vi "init.vi"(0 "Camera in":refnum<class "Camera.lvclass">, 1 "interface":u8(ring)=255 items=["FireWire"=1, "GenICam"=3, "GigE"=5, "USB"=6, "CameraLinkME4"=7, "USB3"=8, "CLHS"=11, "All"=255], 3 "error in (no error)":errorcluster) -> (7 "Camera out":refnum<class "Camera.lvclass">, 10 "error out":errorcluster)   [LabVIEW 2020, in "Camera.lvclass"]
doc: "This function is similar to init.vi but with the additional option to select the interface where\ncameras should be searched for. The default is All Interfaces. In contrast to init.vi, this function\nuses the pco.sdk function PCO_OpenCameraEx.vi to search the interfaces individually.\n\nYou should use this function instead of init.vi when:\n - You want to search for cameras at a specific interface.\n - You want to create multiple Camera objects in an application where the cameras are partially connected during operation."
uses:
  Camera.lvclass
  Camera.lvclass/Camera.ctl
  Structures.lvlib
  CameraAccess.lvlib
  CameraDescription.lvlib
  GeneralCameraStatus.lvlib
  Convert.lvlib
panel:
  out "error out 2":errorcluster {"code" format="%x"}
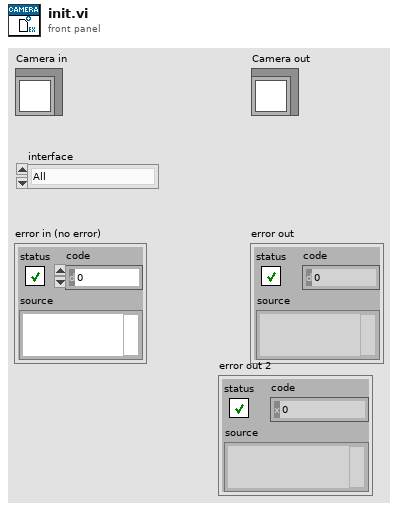
[diagram p1: front panel]
types:
  T1 = cluster{"wCamType":u16, "wCamSubType":u16, "dwSerialNumber":u32, "dwHWVersion":u32, "dwFWVersion":u32, "InterfaceType":u16, "PCO_FW_Vers":cluster{"wDeviceNum":u16, "PCO_SC2_Firmware_DESC":cluster{"szName":string, "bMinorRev":u8, "bMajorRev":u8, "wVariant":u16}[]}, "PCO_HW_Vers":cluster{"wBoardNum":u16, "PCO_SC2_Hardware_DESC":cluster{"szName":string, "wBatchNo":u16, "wRevision":u16, "wVariant":u16}[]}}
  T2 = cluster{"wSensorTypeDESC":u16, "wSensorSubTypeDESC":u16, "wMaxHorzResStdDESC":u16, "wMaxVertResStdDESC":u16, "wMaxHorzResExtDESC":u16, "wMaxVertResExtDESC":u16, "wDynResDESC":u16, "wMaxBinHorzDESC":u16, "wBinHorzSteppingDESC":u16, "wMaxBinVertDESC":u16, "wBinVertSteppingDESC":u16, "wRoiHorStepsDESC":u16, "wRoiVertStepsDESC":u16, "wNumADCsDESC":u16, "wMinSizeHorzDESC":u16, "dwPixelRateDESC":u32[], "wConvFactDESC":u16[], "sCoolingSetpoints":i16[], "wSoftRoiHorStepsDESC":u16, "wSoftRoiVertStepsDESC":u16, "wIRDESC":u16, "wMinSizeVertDESC":u16, "dwMinDelayDESC":u32, "dwMaxDelayDESC":u32, "dwMinDelayStepDESC":u32, "dwMinExposureDESC":u32, "dwMaxExposureDESC":u32, "dwMinExposureStepDESC":u32, "dwMinDelayIRDESC":u32, "dwMaxDelayIRDESC":u32, "dwMinExposureIRDESC":u32, "dwMaxExposureIRDESC":u32, "wTimeTableDESC":u16, "wDoubleImageDESC":u16, "sMinCoolSetDESC":i16, "sMaxCoolSetDESC":i16, "sDefaultCoolSetDESC":i16, "wPowerDownModeDESC":u16, "wOffsetRegulationDESC":u16, "wColorPatternDESC":u16, "wPatternTypeDESC":u16, "wNumCoolingSetpoints":u16, "dwGeneralCapsDESC1":u32, "dwGeneralCapsDESC2":u32, "dwExtSyncFrequency":u32[], "dwGeneralCapsDESC3":u32, "dwGeneralCapsDESC4":u32}
  T3 = cluster{"sharpen":bool, "adaptive_sharpen":bool, "flip_vertical":bool, "auto_minmax":bool, "min_limit":u16, "max_limit":u16, "gamma":dbl, "contrast":i32, "pco_debayer_algorithm":bool, "color_temperature":i32, "color_saturation":i32, "color_vibrance":i32, "color_tint":i32, "lut_file":path}
  T4 = cluster{"wInterfaceType":u16, "wCameraNumber":u16, "wCameraNumAtInterface":u16, "wOpenFlags":u16[], "dwOpenFlags":u32[], "wOpenPtr":u64[]}
  T5 = cluster{"iConversionFactor":i32, "iDataBits":i32, "iSensorInfoBits":i32, "iDarkOffset":i32, "strColorCoeff":dbl[], "iCamNum":i32, "hCamera":u64}
  T6 = enum16{"Undefined", "Mono8", "Mono16", "BGRA8", "RGBA8", "BGRA16", "RGBA16", "CompressedMono8"}
  T7 = map{enum16{"Undefined", "Mono8", "Mono16", "BGRA8", "RGBA8", "BGRA16", "RGBA16", "CompressedMono8"}, bool}
  T8 = map{enum16{"Undefined", "Mono8", "Mono16", "BGRA8", "RGBA8", "BGRA16", "RGBA16", "CompressedMono8"}, cluster{"sharpen":bool, "adaptive_sharpen":bool, "flip_vertical":bool, "auto_minmax":bool, "min_limit":u16, "max_limit":u16, "gamma":dbl, "contrast":i32, "pco_debayer_algorithm":bool, "color_temperature":i32, "color_saturation":i32, "color_vibrance":i32, "color_tint":i32, "lut_file":path}}
  T9 = map{enum16{"Undefined", "Mono8", "Mono16", "BGRA8", "RGBA8", "BGRA16", "RGBA16", "CompressedMono8"}, u64}
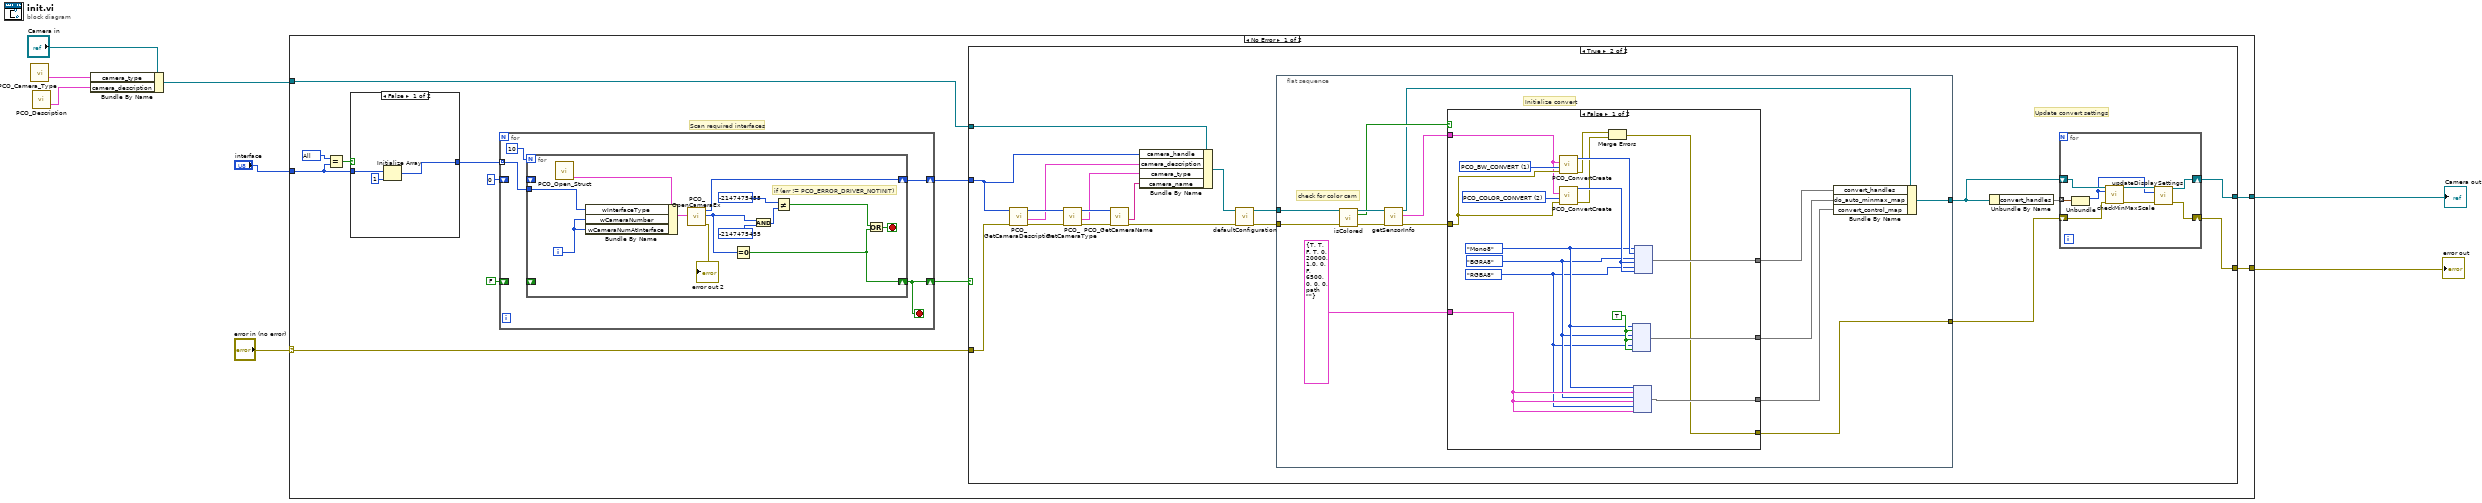
[diagram p0: block diagram]
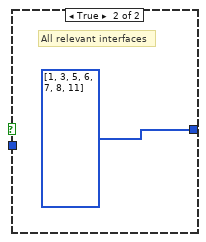
[diagram p2: hidden frame]
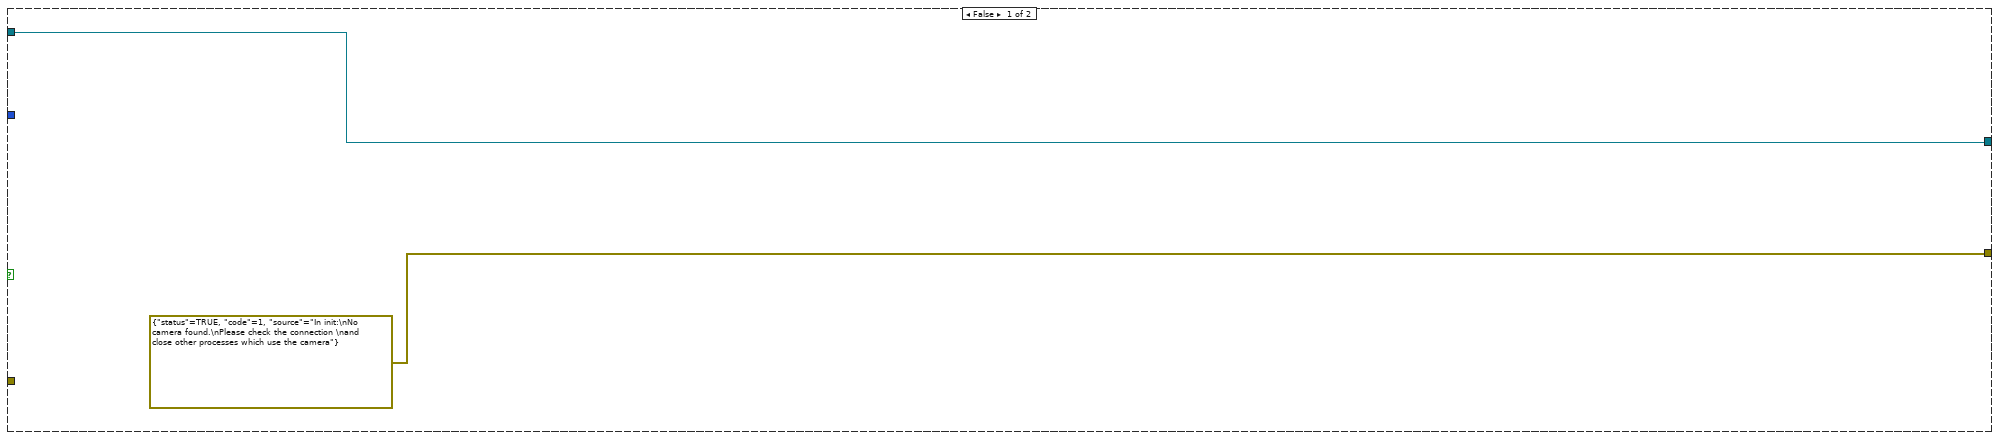
[diagram p3: hidden frame]
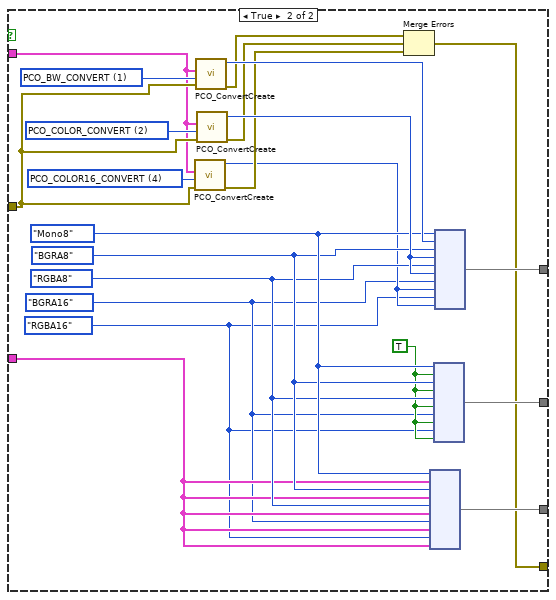
[diagram p4: hidden frame]
diagram:
  n1 = call "PCO_Camera_Type.vi"() -> ("PCO_CameraType"=w4:T1)  [unwired: 4 in, 3 out]
  n2 = call "PCO_Description.vi"() -> ("PCO_Description"=w3:T2)  [unwired: 4 in, 3 out]
  n3 = Bundle By Name(cluster="Camera in", "camera_type"=w4, "camera_description"=w3) -> (w1:refnum<class "Camera.lvclass">)
  n4 = case shown="No Error" "error in (no error)" {
    selector: "error in (no error)" -> [w9 w125]
    tunnel: [w18 w125] -> w7
    tunnel: [w16 w124] -> w6
    tunnel: w1 -> [w17 w124]
    tunnel: "interface" -> [w13 _]
    frame No Error {
      w15 = u8 255 items=["FireWire"=1, "GenICam"=3, "GigE"=5, "USB"=6, "CameraLinkME4"=7, "USB3"=8, "CLHS"=11, "All"=255] ("interface")
      # "Scan required interfaces"
      n5 = Equal?(x=w15, y=w13) -> (x = y?=w14:bool)
      n6 = case shown="False" w14 {
        tunnel: w13 -> [w40 _]
        tunnel: [w38 u8[] [1, 3, 5, 6, 7, 8, 11]] -> w10
        frame False {
          n7 = Initialize Array(w40, 1 ("dimension size")) -> (w38:u8[])
        }
        frame True {
          # "All relevant interfaces"
        }
      }
      n8 = for {
        shift-right: [w23] -> w19
        shift-left: u64 0 ("ph out") -> [_]
        shift-right: [w22] -> w20
        shift-left: FALSE -> [_]
        tunnel: w10 -> [w21] mode=indexing
        stop <- w22 stop-if-true
        n9 = for {
          N: 10 -> [_]
          tunnel: w21 -> [w36]
          shift-right: [w32] -> w22
          shift-left: _ -> [_]
          shift-right: [w30] -> w23
          shift-left: _ -> [_]
          i -> [w26]
          stop <- w31 stop-if-true
          # "if (err != PCO_ERROR_DRIVER_NOTINIT)"
          n10 = call "PCO_Open_Struct.vi"() -> ("PCO_Open_Struct"=w37:T4)  [unwired: 4 in, 4 out]
          n11 = Bundle By Name(cluster=w37, "wInterfaceType"=w36, "wCameraNumber"=w26, "wCameraNumAtInterface"=w26) -> (w35:T4)
          n12 = call "PCO_OpenCameraEx.vi"("strOpenStruct"=w35) -> ("error out"=→"error out 2":errorcluster, "ErrorMessage"=w27:i32, "ph out"=w30:u64)  [unwired: 8 in]
          n13 = Equal To 0?(x=w27) -> (x = 0?=w32:bool)
          n14 = And(x=w27, y=-2147475455 ("x")) -> (x .and. y?=w29:i32)
          n15 = Not Equal?(x=-2147475455, y=w29) -> (x != y?=w33:bool)
          n16 = Or(x=w33, y=w32) -> (x .or. y?=w31:bool)
        }
      }
      n17 = case shown="True" w20 {
        tunnel: [errorcluster {"status"=TRUE, "code"=1, "source"="In init:\nNo camera found.\nPlease check the connection \nand close other processes which use the camera"} ("error out") w45] -> w18
        tunnel: w19 -> [_ w55]
        tunnel: w17 -> [w42 w61]
        tunnel: [w42 w46] -> w16
        tunnel: w9 -> [_ w62]
        frame False {
        }
        frame True {
          # "Update convert settings"
          n18 = call "PCO_GetCameraDescription.vi"("error in (no error)"=w62, "ph"=w55) -> ("error out"=w60:errorcluster, "strDescription"=w56:T2, "ph out"=w59:u64)  [unwired: 6 in, 1 out]
          n19 = call "PCO_GetCameraType.vi"("error in (no error)"=w60, "ph"=w59) -> ("error out"=w57:errorcluster, "strCamType"=w54:T1, "ph out"=w58:u64)  [unwired: 6 in, 1 out]
          n20 = call "PCO_GetCameraName.vi"("error in (no error)"=w57, "ph"=w58) -> ("error out"=w52:errorcluster, "szCameraName"=w53:string)  [unwired: 6 in, 2 out]
          n21 = Bundle By Name(cluster=w61, "camera_handle"=w55, "camera_description"=w56, "camera_type"=w54, "camera_name"=w53) -> (w51:refnum<class "Camera.lvclass">)
          n22 = call-dynamic "defaultConfiguration.vi"("error in (no error)"=w52, "Camera in"=w51) -> ("error out"=w49:errorcluster, "Camera out"=w50:refnum<class "Camera.lvclass">)  [unwired: 8 in]
          n23 = flat-sequence {
            tunnel: w50 -> [w84]
            tunnel: w49 -> [w83]
            tunnel: [w71] -> w47
            tunnel: [w75] -> w44
            frame #0 {
              # "check for color cam"
              # "Initialize convert"
              n24 = call-dynamic "isColored.vi"("Camera in"=w84, "error in (no error)"=w83) -> ("Camera out"=w81:refnum<class "Camera.lvclass">, "colored"=w80:bool, "error out"=w82:errorcluster)  [unwired: 11 in]
              n25 = call-dynamic "getSensorInfo.vi"("error in (no error)"=w82, "Camera in"=w81) -> ("error out"=w77:errorcluster, "PCO_SensorInfo"=w78:T5, "Camera out"=w76:refnum<class "Camera.lvclass">)  [unwired: 7 in]
              n26 = case shown="False" w80 {
                tunnel: [w100 w111] -> w74
                tunnel: [w101 w104] -> w73
                tunnel: T3 {"sharpen"=TRUE, "adaptive_sharpen"=TRUE, "flip_vertical"=FALSE, "auto_minmax"=TRUE, "min_limit"=0, "max_limit"=20000, "gamma"=1.0, "contrast"=0, "pco_debayer_algorithm"=FALSE, "color_temperature"=6500, "color_saturation"=0, "color_vibrance"=0, "color_tint"=0, "lut_file"=path ""} ("convert_control") -> [w98 w110]
                tunnel: [w99 w103] -> w72
                tunnel: w78 -> [w93 w112]
                tunnel: w77 -> [w94 w113]
                tunnel: [w85 w102] -> w71
                frame False {
                  w86 = T6."RGBA8" ("data_format")
                  w87 = T6."BGRA8" ("data_format")
                  w88 = T6."Mono8" ("data_format")
                  w97 = TRUE
                  w95 = 2 items=["PCO_BW_CONVERT"=1, "PCO_COLOR_CONVERT"=2, "PCO_PSEUDO_CONVERT"=3, "PCO_COLOR16_CONVERT"=4]
                  w96 = 1 items=["PCO_BW_CONVERT"=1, "PCO_COLOR_CONVERT"=2, "PCO_PSEUDO_CONVERT"=3, "PCO_COLOR16_CONVERT"=4]
                  n27 = call "PCO_ConvertCreate.vi"("error in (no error)"=w94, "iConvertType"=w96, "strSensor"=w93) -> ("error out"=w90:errorcluster, "ph out"=w92:u64)  [unwired: 6 in, 1 out]
                  n28 = call "PCO_ConvertCreate.vi"("error in (no error)"=w94, "iConvertType"=w95, "strSensor"=w93) -> ("error out"=w89:errorcluster, "ph out"=w91:u64)  [unwired: 6 in, 1 out]
                  n29 = Merge Errors(w90, w89) -> (w85:errorcluster)
                  n30 = node(w88, w97, w87, w97, w86, w97) -> (w101:T7)
                  n31 = node(w88, w98, w87, w98, w86, w98) -> (w99:T8)
                  n32 = node(w88, w92, w87, w91, w86, w91) -> (w100:T9)
                }
                frame True {
                  w105 = T6."RGBA16" ("data_format")
                  w106 = T6."BGRA16" ("data_format")
                  w114 = 4 items=["PCO_BW_CONVERT"=1, "PCO_COLOR_CONVERT"=2, "PCO_PSEUDO_CONVERT"=3, "PCO_COLOR16_CONVERT"=4]
                  w115 = T6."RGBA8" ("data_format")
                  w116 = T6."BGRA8" ("data_format")
                  w117 = T6."Mono8" ("data_format")
                  w109 = TRUE
                  w122 = 2 items=["PCO_BW_CONVERT"=1, "PCO_COLOR_CONVERT"=2, "PCO_PSEUDO_CONVERT"=3, "PCO_COLOR16_CONVERT"=4]
                  w123 = 1 items=["PCO_BW_CONVERT"=1, "PCO_COLOR_CONVERT"=2, "PCO_PSEUDO_CONVERT"=3, "PCO_COLOR16_CONVERT"=4]
                  n33 = call "PCO_ConvertCreate.vi"("error in (no error)"=w113, "iConvertType"=w114, "strSensor"=w112) -> ("error out"=w108:errorcluster, "ph out"=w107:u64)  [unwired: 6 in, 1 out]
                  n34 = call "PCO_ConvertCreate.vi"("error in (no error)"=w113, "iConvertType"=w123, "strSensor"=w112) -> ("error out"=w119:errorcluster, "ph out"=w121:u64)  [unwired: 6 in, 1 out]
                  n35 = call "PCO_ConvertCreate.vi"("error in (no error)"=w113, "iConvertType"=w122, "strSensor"=w112) -> ("error out"=w118:errorcluster, "ph out"=w120:u64)  [unwired: 6 in, 1 out]
                  n36 = Merge Errors(w119, w118, w108) -> (w102:errorcluster)
                  n37 = node(w117, w110, w116, w110, w115, w110, w106, w110, w105, w110) -> (w103:T8)
                  n38 = node(w117, w109, w116, w109, w115, w109, w106, w109, w105, w109) -> (w104:T7)
                  n39 = node(w117, w121, w116, w120, w115, w120, w106, w107, w105, w107) -> (w111:T9)
                }
              }
              n40 = Bundle By Name(cluster=w76, "convert_handles"=w74, "do_auto_minmax_map"=w73, "convert_control_map"=w72) -> (w75:refnum<class "Camera.lvclass">)
            }
          }
          n41 = Unbundle By Name(w44) -> ("convert_handles"=w48:T9)
          n42 = for {
            tunnel: w48 -> [w70] mode=indexing
            shift-right: [w69] -> w46
            shift-left: w44 -> [w67]
            shift-right: [w68] -> w45
            shift-left: w47 -> [w65]
            n43 = Unbundle(w70) -> (w63:T6)  [unwired: 1 out]
            n44 = call-dynamic "checkMinMaxScale.vi"("Camera in"=w67, "data_format"=w63, "error in (no error)"=w65) -> ("Camera out"=w66:refnum<class "Camera.lvclass">, "error out"=w64:errorcluster)  [unwired: 10 in, 1 out]
            n45 = call-dynamic "updateDisplaySettings.vi"("Camera in"=w66, "data_format"=w63, "error in (no error)"=w64) -> ("Camera out"=w69:refnum<class "Camera.lvclass">, "error out"=w68:errorcluster)  [unwired: 11 in]
          }
        }
      }
    }
    frame Error {
    }
  }
  "error out" <- w7
  "Camera out" <- w6
